vi "Init Device.vi"(7 "Layout Ref":refnum<vi>, 8 "error in (no error)":errorcluster, 10 "Chan# Array":i32[](array[numeric]), 11 "Arduino DDS in":refnum<class "Arduino DDS.lvclass">) -> (0 "error out":errorcluster, 3 "Arduino DDS out":refnum<class "Arduino DDS.lvclass">)   [LabVIEW 2013, in "Arduino DDS.lvclass"]
doc: "Initialize the correct columns and their default appearance.\nUse the front panel to change default appearance of the device in the Add/Manage devices.\n\nOpen a specific device implementation for details."
uses:
  Arduino DDS.lvclass
  TypeDefs/ColumnAppearCluster.ctl
  TypeDefs/DigitalColumnAppearCluster.ctl
  ColumnVIs/Column/Column.lvclass
  ColumnVIs/DigitalCol/DigitalCol.lvclass
panel:
  in  "Freq_F":T1={"Column Name"="", "Width"=30, "Bkgd"=[16448250], "Text"=[0]}
  in  "Phase":T1={"Column Name"="", "Width"=30, "Bkgd"=[16448250], "Text"=[0]}
  in  "Sweep?":T2={"Column Name"="", "Width"=15, "Bkgd"=[1985280, 6618880, 14090026], "Text"=[16448250, 0, 0]}
  in  "Freq_I":T1={"Column Name"="", "Width"=30, "Bkgd"=[16448250], "Text"=[0]}
  # "Open a specific devices override of this VI for implementation."
  # "Intended functionality:\n------------------------\nPlace controls here for Device programmer OR advanced user to configure\ntypical layout in the table.\n\nDisplay Info.vi (called on add/manage device) will be where typical user can fine tune."
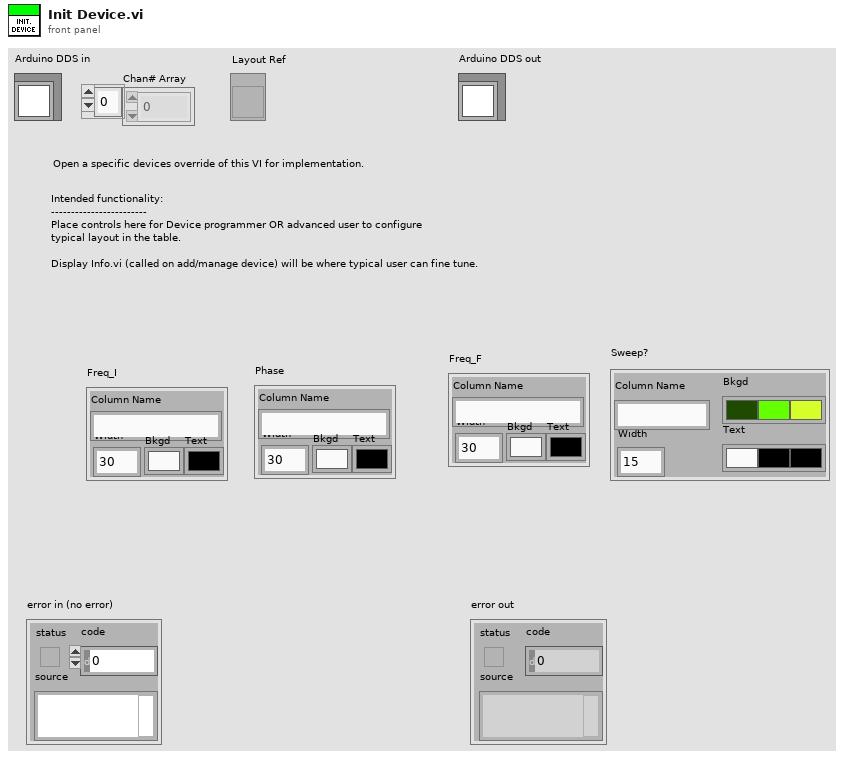
[diagram p1: front panel]
types:
  T1 = typedef "ColumnAppearCluster.ctl" = cluster{"Column Name":string, "Width":u32, "Bkgd":u32[], "Text":u32[]}
  T2 = typedef "DigitalColumnAppearCluster.ctl" = cluster{"Column Name":string, "Width":u32, "Bkgd":u32[], "Text":u32[]}
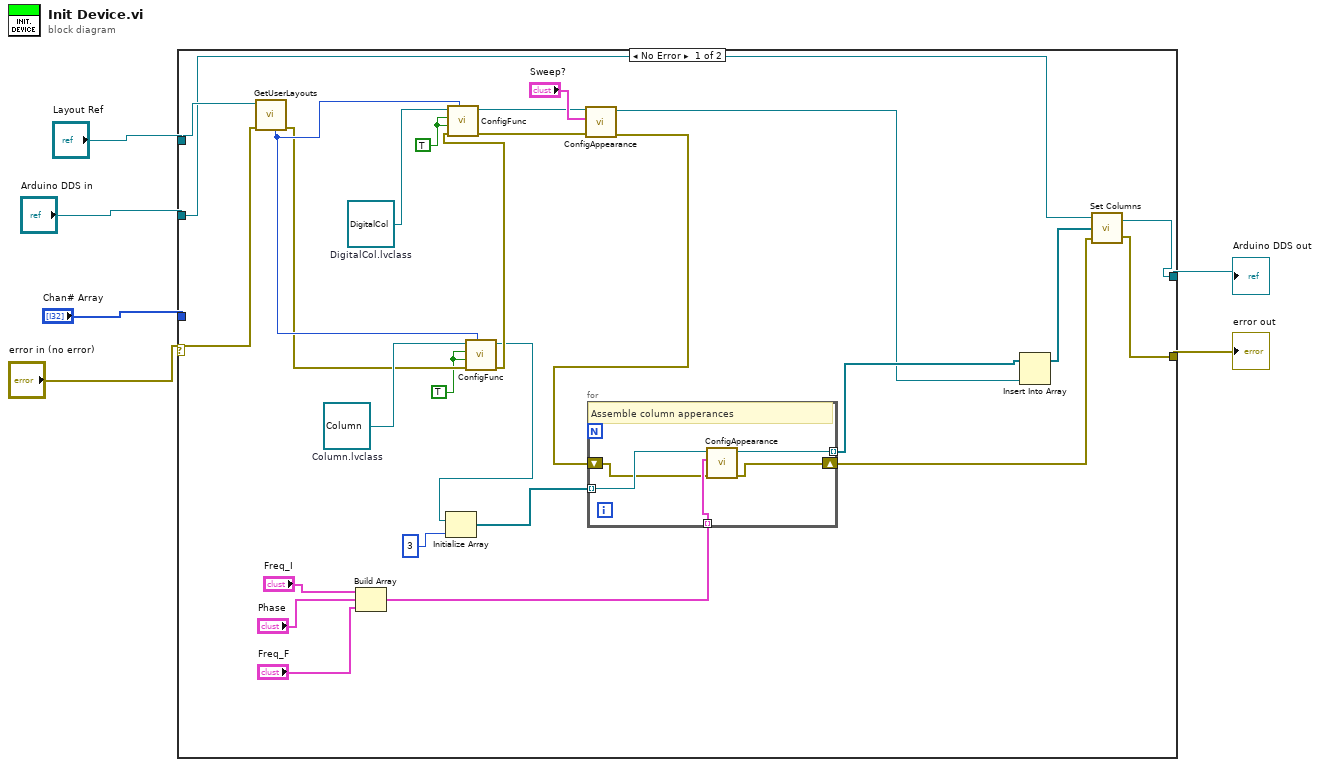
[diagram p0: block diagram]
diagram:
  n1 = case shown="No Error" "error in (no error)" {
    selector: "error in (no error)" -> [w32 w40]
    tunnel: [w8 w40] -> w5
    tunnel: "Arduino DDS in" -> [w7 w39]
    tunnel: [w10 w39] -> w3
    tunnel: "Chan# Array" -> [_ _]
    tunnel: "Layout Ref" -> [w33 _]
    frame No Error {
      w26 = TRUE ("Disableable? (True)")
      w25 = TRUE ("Disableable? (True)")
      w30 = refnum<class "DigitalCol.lvclass"> refnum  # DigitalCol.lvclass
      w29 = refnum<class "Column.lvclass"> refnum  # Column.lvclass
      n2 = call "GetUserLayouts.vi"("error in (no error)"=w32, "Layout Ring Refnum"=w33) -> ("error out"=w28:errorcluster, "Num User Layouts"=w31:i32)  [unwired: 5 in, 3 out]
      n3 = Build Array("Freq_I", "Phase", "Freq_F") -> (w18:T1[])
      n4 = call "ConfigFunc.vi"("Num Layouts (ignored)"=w31, "error in (no error)"=w28, "isVariable? (True)"=w26, "Disableable? (True)"=w26, "Column in"=w29) -> ("error out"=w27:errorcluster, "Column out"=w16:refnum<class "Column.lvclass">)  [unwired: 5 in]
      n5 = Initialize Array(w16, 3) -> (w15:refnum<class "Column.lvclass">[])
      n6 = call "ConfigFunc.vi"("Num Layouts (ignored)"=w31, "error in (no error)"=w27, "isVariable? (True)"=w25, "Disableable? (True)"=w25, "Column in"=w30) -> ("error out"=w24:errorcluster, "Column out"=w22:refnum<class "DigitalCol.lvclass">)  [unwired: 5 in]
      n7 = call "ConfigAppearance.vi"("error in (no error)"=w24, "Column Appearance"="Sweep?", "Column in"=w22) -> ("error out"=w14:errorcluster, "Column out"=w12:refnum<class "DigitalCol.lvclass">)  [unwired: 7 in]
      n8 = for {
        tunnel: w18 -> [w38] mode=indexing
        tunnel: w15 -> [w37] mode=indexing
        shift-right: [w35] -> w9
        shift-left: w14 -> [w36]
        tunnel: [w34] -> w13 mode=indexing
        # "Assemble column apperances"
        n9 = call "ConfigAppearance.vi"("error in (no error)"=w36, "Column Appearance"=w38, "Column in"=w37) -> ("error out"=w35:errorcluster, "Column out"=w34:refnum<class "Column.lvclass">)  [unwired: 7 in]
      }
      n10 = Insert Into Array(array=w13, new element=w12) -> (w11:refnum<class "Column.lvclass">[])  [unwired: 1 in]
      n11 = call-dynamic "Set Columns.vi"("error in (no error)"=w9, "Columns"=w11, "Arduino DDS in"=w7) -> ("error out"=w8:errorcluster, "Arduino DDS out"=w10:refnum<class "Arduino DDS.lvclass">)  [unwired: 1 in]
    }
    frame Error {
    }
  }
  "error out" <- w5
  "Arduino DDS out" <- w3
